vi "irqTest.vi"() -> ()   [LabVIEW 2016]
uses:
  <vilib>/FPGAPlugInAG/cRIO-9038/niLvFpga_Open_cRIO-9038.vi
  <vilib>/rvi/interface/common/dynamic/niFpgaDynamicAddResources.vi
  <vilib>/FPGAPlugInAG/Dynamic/niLvFpga_Abort_Dynamic.vi
  <vilib>/FPGAPlugInAG/Dynamic/niLvFpga_Reset_Dynamic.vi
  <vilib>/FPGAPlugInAG/Dynamic/niLvFpga_Run_Dynamic.vi
  <vilib>/Utility/error.llb/Error Cluster From Error Code.vi
  <vilib>/RVI Host/nirviSupport.llb/nirviErrorClusterFromErrorCode.vi
  <vilib>/rvi/errors/niLvFpgaAdjustHostInterfaceError.vi
  <vilib>/rvi/interface/nirviOpenFPGA/nirviOpenFPGA.xnode
  FPGA Bitfiles/Modbus_FPGATarget_irqTest_EsivkxyOnps.lvbitx
  <vilib>/rvi/interface/nirviMethod/nirviMethod.xnode
  <vilib>/rvi/interface/nirviMethod/StockFPGA_InlinedMethodWaitForSingleIRQ.vi
  <vilib>/FPGAPlugInAG/Dynamic/niLvFpga_WaitOnIrq_Dynamic.vi
  <vilib>/rvi/interface/nirviMethod/StockFPGA_InlinedMethodWaitForMultipleIRQ.vi
  <vilib>/FPGAPlugInAG/Dynamic/niLvFpga_AcknowledgeIrq_Dynamic.vi
panel:
  in  "Boolean 3":bool
  out "IRQ2-3":i32
  in  "Boolean 2":bool
  out "IRQ1":i32
  out "IRQ0":i32
  in  "Boolean":bool
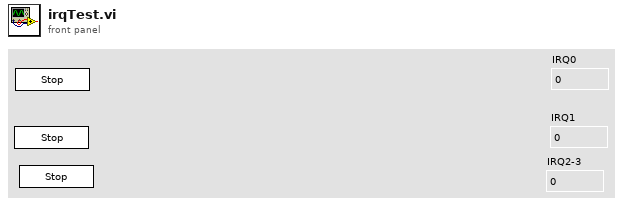
[diagram p1: front panel]
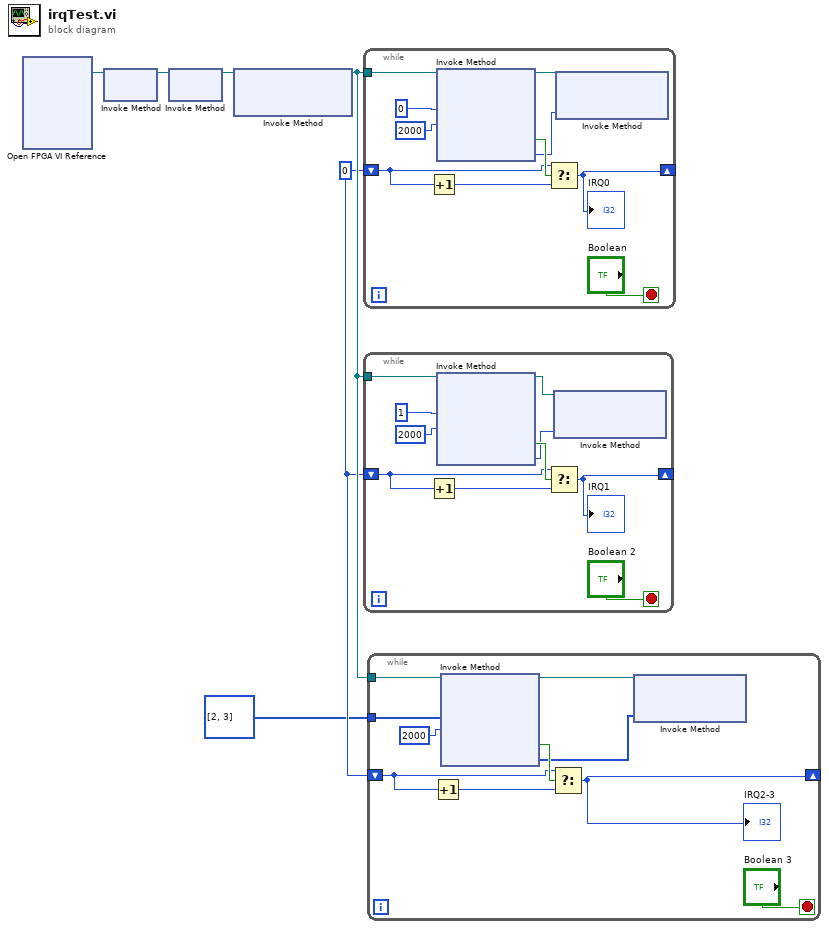
[diagram p0: block diagram]
diagram:
  w2 = 0
  n1 = xnode "Open FPGA VI Reference"() -> ("FPGA VI Reference Out"=w6:refnum<k20>)  [unwired: 2 in, 1 out]
  n2 = xnode "Invoke Method"("FPGA VI Reference In"=w6) -> ("FPGA VI Reference Out"=w5:refnum<k20>)  [unwired: 1 in, 1 out]
  n3 = xnode "Invoke Method"("FPGA VI Reference In"=w5) -> ("FPGA VI Reference Out"=w4:refnum<k20>)  [unwired: 1 in, 1 out]
  n4 = xnode "Invoke Method"("FPGA VI Reference In"=w4) -> ("FPGA VI Reference Out"=w3:refnum<k20>)  [unwired: 2 in, 1 out]
  n5 = while {
    tunnel: w3 -> [w15]
    shift-right: [w9] -> _
    shift-left: w2 -> [w11]
    stop <- "Boolean" stop-if-true
    n6 = Increment(x=w11) -> (x+1=w10:i32)
    n7 = xnode "Invoke Method"("FPGA VI Reference In"=w15, "IRQ Number(s)"=0, "Timeout (ms)"=2000) -> ("FPGA VI Reference Out"=w8:refnum<k20>, "Timed Out"=w12:bool, "IRQ(s) Asserted"=w7:i32)  [unwired: 1 in, 1 out]
    n8 = Select(t=w11, s=w12, f=w10) -> (s? t:f=w9:i32)
    "IRQ0" <- w9
    n9 = xnode "Invoke Method"("FPGA VI Reference In"=w8, "IRQ Number(s)"=w7) -> ()  [unwired: 1 in, 2 out]
  }
  n10 = while {
    tunnel: w3 -> [w25]
    shift-right: [w19] -> _
    shift-left: w2 -> [w21]
    stop <- "Boolean 2" stop-if-true
    n11 = Increment(x=w21) -> (x+1=w20:i32)
    n12 = xnode "Invoke Method"("FPGA VI Reference In"=w25, "IRQ Number(s)"=1, "Timeout (ms)"=2000) -> ("FPGA VI Reference Out"=w18:refnum<k20>, "Timed Out"=w22:bool, "IRQ(s) Asserted"=w17:i32)  [unwired: 1 in, 1 out]
    n13 = Select(t=w21, s=w22, f=w20) -> (s? t:f=w19:i32)
    "IRQ1" <- w19
    n14 = xnode "Invoke Method"("FPGA VI Reference In"=w18, "IRQ Number(s)"=w17) -> ()  [unwired: 1 in, 2 out]
  }
  n15 = while {
    tunnel: w3 -> [w35]
    shift-right: [w30] -> _
    shift-left: w2 -> [w32]
    tunnel: i32[] [2, 3] -> [w29]
    stop <- "Boolean 3" stop-if-true
    n16 = Increment(x=w32) -> (x+1=w31:i32)
    n17 = xnode "Invoke Method"("FPGA VI Reference In"=w35, "IRQ Number(s)"=w29, "Timeout (ms)"=2000) -> ("FPGA VI Reference Out"=w28:refnum<k20>, "Timed Out"=w33:bool, "IRQ(s) Asserted"=w27:i32[])  [unwired: 1 in, 1 out]
    n18 = Select(t=w32, s=w33, f=w31) -> (s? t:f=w30:i32)
    "IRQ2-3" <- w30
    n19 = xnode "Invoke Method"("FPGA VI Reference In"=w28, "IRQ Number(s)"=w27) -> ()  [unwired: 1 in, 2 out]
  }
